vi "Main.vi"   [LabVIEW 2024, in "Application.lvlib"]
uses:
  Application.lvlib
  Support/User Events/User Events - Create.vi
  Support/User Events/User Events - Destroy.vi
  Support/User Events/User Events.lvlib
  Modules/User Interface/User Interface.lvlib
  Modules/Session Scanner/Session Scanner.lvlib
  Modules/Data Base/Data Base.lvlib
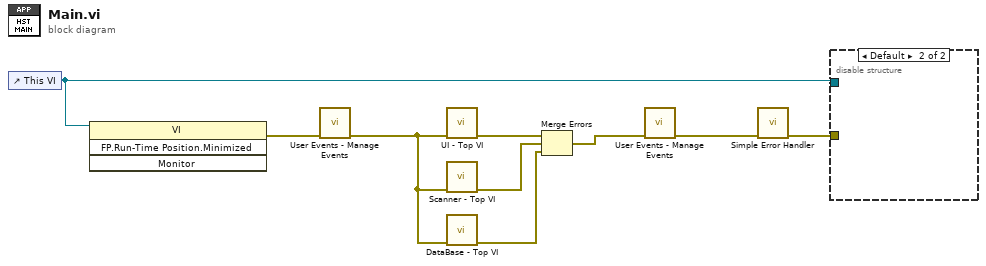
[diagram p0: block diagram]
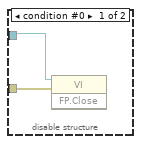
[diagram p2: hidden frame]
diagram:
  n1 = control-ref of="This VI"() -> (w2:refnum<vi>)
  n2 = invoke class="VI" method="FP.Run-Time Position.Minimized"(reference=w2) -> (error out=w3:errorcluster)  [unwired: 3 in, 3 out]
  n3 = call-poly "User Events - Manage Events.vi"("error in"=w3) -> ("error out"=w5:errorcluster)  [unwired: 10 in]
  n4 = call "UI - Top VI.vi"("error in"=w5) -> ("error out"=w9:errorcluster)  [unwired: 10 in]
  n5 = call "Scanner - Top VI.vi"("error in"=w5) -> ("error out"=w6:errorcluster)  [unwired: 10 in]
  n6 = call "DataBase - Top VI.vi"("error in"=w5) -> ("error out"=w4:errorcluster)  [unwired: 10 in]
  n7 = Merge Errors(w9, w6, w4) -> (w7:errorcluster)
  n8 = call-poly "User Events - Manage Events.vi"("error in"=w7) -> ("error out"=w8:errorcluster)  [unwired: 10 in]
  n9 = call <vilib>:"Simple Error Handler.vi"("error in (no error)"=w8) -> ("error out"=w1:errorcluster)  [unwired: 4 in, 4 out]
  n10 = disable-structure shown="Default" {
    disable-tunnel: w2 -> [w11 _]
    disable-tunnel: w1 -> [w10 _]
    frame condition #0 {
      n11 = invoke class="VI" method="FP.Close"(reference=w11, error in=w10) -> ()  [unwired: 1 in, 3 out]
    }
    frame condition #1 (active) {
    }
  }
